vi "execute.vi"(8 "error in (no error)":errorcluster, 9 "image assembler in":refnum<class "GenericComponent.lvclass">, 10 "trajectory in":refnum<class "GenericComponent.lvclass">, 11 "DL090521TrajectoryToImageAssemblerAdapter in":refnum<class "AdapterDL090521TrajectoryToImageAssembler.lvclass">) -> (0 "error out":errorcluster, 1 "image assembler out":refnum<class "GenericComponent.lvclass">, 2 "trajectory out":refnum<class "GenericComponent.lvclass">, 3 "DL090521TrajectoryToImageAssemblerAdapter out":refnum<class "AdapterDL090521TrajectoryToImageAssembler.lvclass">)   [LabVIEW 2010, in "AdapterDL090521TrajectoryToImageAssembler.lvclass"]
uses:
  AdapterDL090521TrajectoryToImageAssembler.lvclass
  common/classes/GenericComponent/GenericComponent/GenericComponent.lvclass
  Trajectory/TrajectoryDL090201FrameScan/TrajectoryDL090201FrameScan/TrajectoryDL090201FrameScan.lvclass
  common/enumerations/unit.ctl
  ImageAssembler/ImageAssemblerDL090211Frame/ImageAssemblerDL090211Frame/ImageAssemblerDL090211Frame.lvclass
  common/classes/Box/Box/Box.lvclass
  common/classes/SpaceVector/SpaceVector/SpaceVector.lvclass
  common/classes/Image/Image/Image.lvclass
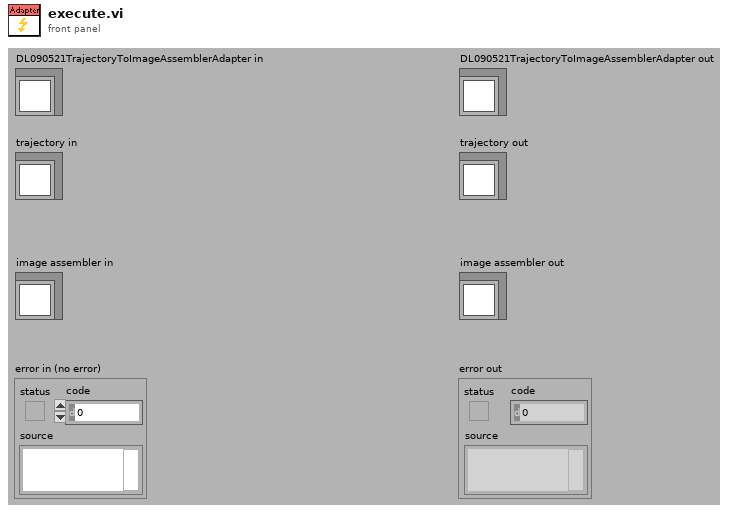
[diagram p1: front panel]
types:
  T1 = typedef "Image.lvclass/unit.ctl" = enum16{"um", "s"}
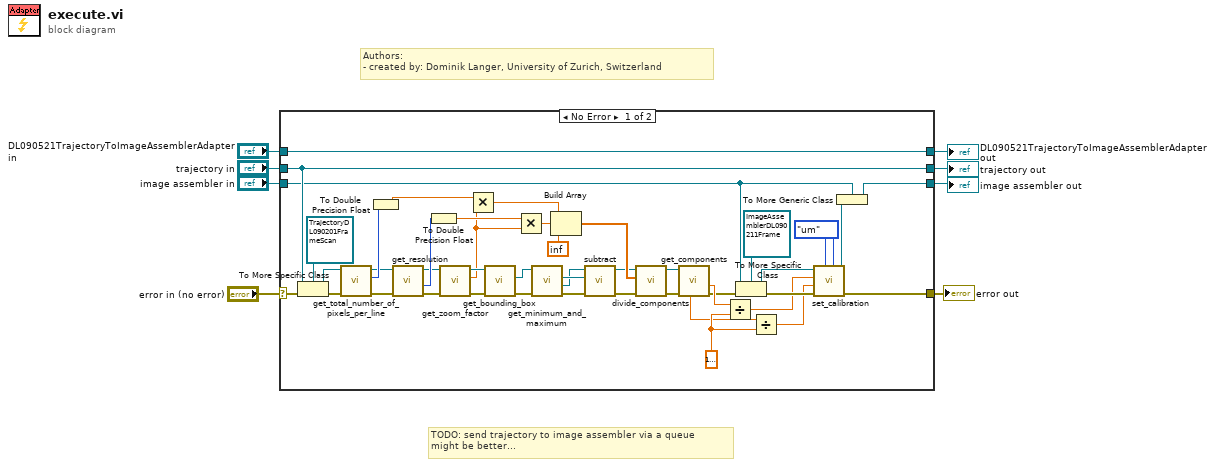
[diagram p0: block diagram]
diagram:
  # "TODO: send trajectory to image assembler via a queue\nmight be better..."
  # "Authors: \n- created by: Dominik Langer, University of Zurich, Switzerland"
  n1 = case shown="No Error" "error in (no error)" {
    selector: "error in (no error)" -> [w51 w55]
    tunnel: "DL090521TrajectoryToImageAssemblerAdapter in" -> [w52 w56]
    tunnel: [w52 w56] -> w6
    tunnel: [w26 w55] -> w5
    tunnel: "trajectory in" -> [w50 w54]
    tunnel: "image assembler in" -> [w23 w53]
    tunnel: [w50 w54] -> w2
    tunnel: [w22 w53] -> w1
    frame No Error {
      w19 = unit."um" ("x unit")
      w32 = dbl[unit] 1e-06 ("y")
      n2 = To More Specific Class(target class=refnum<class "TrajectoryDL090201FrameScan.lvclass"> refnum ("TrajectoryDL090201FrameScan.lvclass"), reference=w50, error in=w51) -> (specific class reference=w35:refnum<class "TrajectoryDL090201FrameScan.lvclass">, error out=w39:errorcluster)
      n3 = call-dynamic "get_total_number_of_pixels_per_line.vi"("error in (no error)"=w39, "DL090201FrameScanTrajectory in"=w35) -> ("error out"=w37:errorcluster, "total number of pixels per line"=w38:i32, "DL090201FrameScanTrajectory out"=w36:refnum<class "TrajectoryDL090201FrameScan.lvclass">)  [unwired: 7 in]
      n4 = To Double Precision Float(number=w38) -> (double precision float=w14:dbl)
      n5 = call-dynamic "get_resolution.vi"("error in (no error)"=w37, "TrajectoryDL090201FrameScan in"=w36) -> ("error out"=w18:errorcluster, "y"=w42:i32, "TrajectoryDL090201FrameScan out"=w17:refnum<class "TrajectoryDL090201FrameScan.lvclass">)  [unwired: 7 out]
      n6 = To Double Precision Float(number=w42) -> (double precision float=w13:dbl)
      n7 = call-dynamic "get_zoom_factor.vi"("error in (no error)"=w18, "GenericTrajectory in"=w17) -> ("error out"=w16:errorcluster, "current zoom factor"=w11:dbl, "GenericTrajectory out"=w15:refnum<class "TrajectoryDL090201FrameScan.lvclass">)  [unwired: 7 out]
      n8 = Multiply(x=w14, y=w11) -> (x*y=w12:dbl)
      n9 = call-dynamic "get_bounding_box.vi"("error in (no error)"=w16, "GenericTrajectory in"=w15) -> ("error out"=w49:errorcluster, "Box.lvclass"=w48:refnum<class "Box.lvclass">)  [unwired: 7 in, 1 out]
      n10 = Multiply(x=w13, y=w11) -> (x*y=w10:dbl)
      n11 = call "get_minimum_and_maximum.vi"("error in (no error)"=w49, "Box in"=w48) -> ("error out"=w47:errorcluster, "maximum"=w45:refnum<class "SpaceVector.lvclass">, "minimum"=w46:refnum<class "SpaceVector.lvclass">)  [unwired: 7 out]
      n12 = Build Array(w12, w10, inf) -> (w43:dbl[])
      n13 = call "subtract.vi"("error in (no error)"=w47, "subtrahend"=w46, "SpaceVector in"=w45) -> ("error out"=w41:errorcluster, "SpaceVector out"=w40:refnum<class "SpaceVector.lvclass">)  [unwired: 7 out]
      n14 = call "divide_components.vi"("error in (no error)"=w41, "divisors"=w43, "SpaceVector in"=w40) -> ("error out"=w34:errorcluster, "SpaceVector out"=w33:refnum<class "SpaceVector.lvclass">)  [unwired: 7 out]
      n15 = call "get_components.vi"("error in (no error)"=w34, "SpaceVector in"=w33) -> ("error out"=w29:errorcluster, "x"=w31:dbl[unit], "y"=w30:dbl[unit])  [unwired: 7 out]
      n16 = Divide(x=w31, y=w32) -> (x/y=w21:dbl)
      n17 = To More Specific Class(target class=refnum<class "ImageAssemblerDL090211Frame.lvclass"> refnum ("DL090211FrameImageAssembler.lvclass"), reference=w23, error in=w29) -> (specific class reference=w25:refnum<class "ImageAssemblerDL090211Frame.lvclass">, error out=w27:errorcluster)
      n18 = Divide(x=w30, y=w32) -> (x/y=w20:dbl)
      n19 = call-dynamic "set_calibration.vi"("y unit"=w19, "x unit"=w19, "error in (no error)"=w27, "y"=w20, "x"=w21, "DL090211ImageAssemblerScaffold in"=w25) -> ("error out"=w26:errorcluster, "DL090211ImageAssemblerScaffold out"=w24:refnum<class "ImageAssemblerDL090211Frame.lvclass">)  [unwired: 4 out]
      n20 = To More Generic Class(target class=w23, reference=w24) -> (generic class reference=w22:refnum<class "GenericComponent.lvclass">)
    }
    frame Error {
    }
  }
  "error out" <- w5
  "DL090521TrajectoryToImageAssemblerAdapter out" <- w6
  "image assembler out" <- w1
  "trajectory out" <- w2
